vi "Extract encoder values from file.vi"() -> ()   [LabVIEW 2018]
panel:
  out "# lines":i32
  in  "file name":string
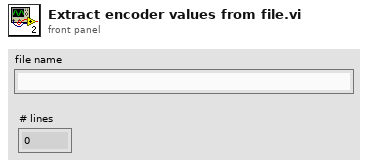
[diagram p1: front panel]
types:
  T1 = enum16{"open", "replace", "create", "open or create", "replace or create", "replace or create with confirmation"}
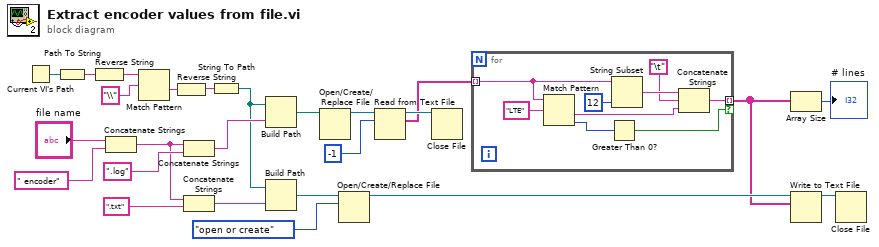
[diagram p0: block diagram]
diagram:
  n1 = Current VI's Path() -> (path=w22:path)
  n2 = Path To String(path=w22) -> (string=w21:string)
  n3 = Reverse String(1:w21) -> (0:w20:string)
  n4 = Concatenate Strings("file name", " encoder" ("string")) -> (w1:string)
  n5 = Match Pattern(string=w20, regular expression="\\") -> (after substring=w24:string)  [unwired: 1 in, 3 out]
  n6 = Reverse String(1:w24) -> (0:w23:string)
  n7 = Concatenate Strings(w1, ".log" ("regular expression")) -> (w19:string)
  n8 = Concatenate Strings(w1, ".txt" ("regular expression")) -> (w18:string)
  n9 = String To Path(string=w23) -> (path=w17:path)
  n10 = Build Path(base path=w17, name or relative path=w19) -> (appended path=w9:path)
  n11 = Build Path(base path=w17, name or relative path=w18) -> (appended path=w14:path)
  n12 = Open/Create/Replace File(file path (use dialog)=w9) -> (refnum out=w12:refnum<file>)  [unwired: 5 in, 2 out]
  n13 = Open/Create/Replace File(file path (use dialog)=w14, operation (0:open)=T1."open or create") -> (refnum out=w7:refnum<file>)  [unwired: 4 in, 2 out]
  n14 = Read from Text File(file (use dialog)=w12, count=-1) -> (refnum out=w11:refnum<file>, text=w8:string[])  [unwired: 2 in, 2 out]
  n15 = Close File(refnum=w11) -> ()  [unwired: 1 in, 2 out]
  n16 = for {
    tunnel: w8 -> [w33] mode=indexing
    tunnel: [w29] -> w5 mode=indexing if=w26
    n17 = Match Pattern(string=w33, regular expression="LTE") -> (after substring=w30:string, offset past match=w27:i32)  [unwired: 1 in, 2 out]
    n18 = Greater Than 0?(x=w27) -> (x > 0?=w26:bool)
    n19 = String Subset(string=w33, length (rest)=12 ("length (rest)")) -> (substring=w32:string)  [unwired: 1 in]
    n20 = Concatenate Strings(w32, "\t", w30) -> (w29:string)
  }
  n21 = Array Size(array=w5) -> (size(s)=→"# lines":i32)
  n22 = Write to Text File(file (use dialog)=w7, text=w5) -> (refnum out=w6:refnum<file>)  [unwired: 2 in, 2 out]
  n23 = Close File(refnum=w6) -> ()  [unwired: 1 in, 2 out]
